vi "sub_InitDevices.vi"(8 "error in (no error)":errorcluster, 10 "Dynamic data":T1, 11 "Input parameters":T2={"Measurement type"=enum."Test", "Sensor type"=enum."One channel", "Input file"="", "Output file"="test.txt", "Open after execution?"=FALSE, "Display channel"=0, "Voltage Delay (s)"=0.5, "Switch Delay (s)"=0.01, "VISA resource name source"="", "VISA resource name LCR"="", "Voltage Limit (V)"=1000.0, "Enable Voltage Auto Range (T:Enable)"=TRUE, "Voltage Manual Range (1.0)"=1.0, "Compliance  Level (uA)"=10.0} {"Voltage Limit (V)" format="%#_13g"; "Voltage Delay (s)" format="%#_13g"; "Switch Delay (s)" format="%#_13g"}) -> (0 "error out":errorcluster, 2 "Dynamic data":T1, 3 "Input parameters":T2={"Measurement type"=enum."Test", "Sensor type"=enum."One channel", "Input file"="", "Output file"="test.txt", "Open after execution?"=FALSE, "Display channel"=0, "Voltage Delay (s)"=0.5, "Switch Delay (s)"=0.01, "VISA resource name source"="", "VISA resource name LCR"="", "Voltage Limit (V)"=1000.0, "Enable Voltage Auto Range (T:Enable)"=TRUE, "Voltage Manual Range (1.0)"=1.0, "Compliance  Level (uA)"=10.0} {"Voltage Limit (V)" format="%#_13g"; "Voltage Delay (s)" format="%#_13g"; "Switch Delay (s)" format="%#_13g"})   [LabVIEW 2015]
uses:
  Program Files (x86)/National Instruments/LabVIEW 2016/instr.lib/Keithley 24XX/Keithley 24XX.lvlib
  Input_parameters.ctl
  Dynamic_data.ctl
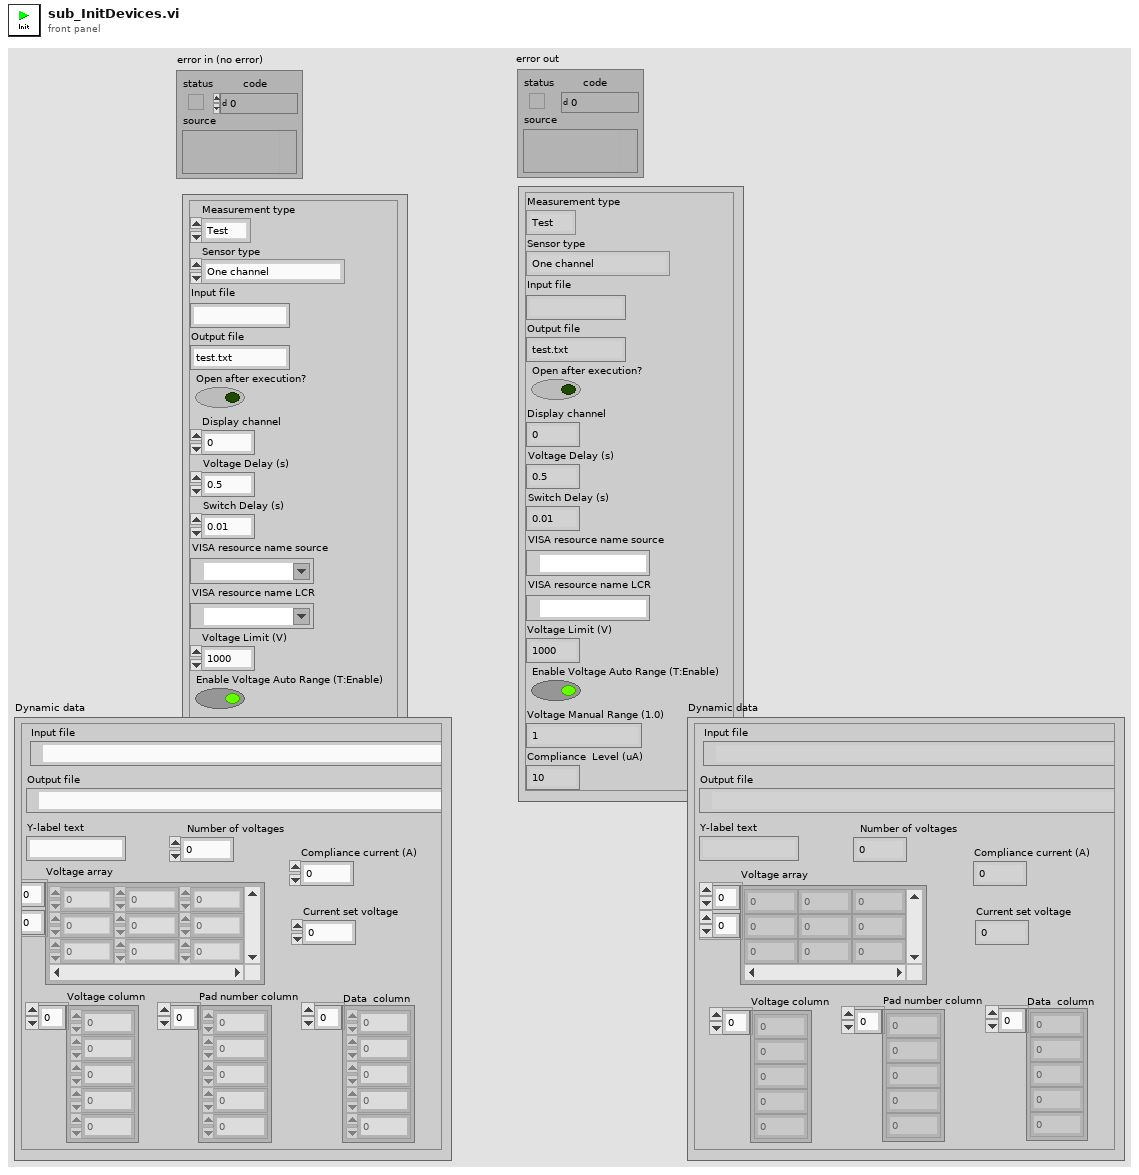
[diagram p1: front panel]
types:
  T1 = typedef "Dynamic_data.ctl" = cluster{"Input file":path, "Output file":path, "Y-label text":string, "Voltage array":dbl[][], "Current set voltage":dbl, "Voltage column":dbl[], "Pad number column":dbl[], "Data  column":dbl[], "Number of voltages":i32, "Compliance current (A)":dbl}
  T2 = typedef "Input_parameters.ctl" = cluster{"Measurement type":enum16{"IV", "CV", "Test"}, "Sensor type":enum16{"6''", "8''", "One channel"}, "Input file":string, "Output file":string, "Open after execution?":bool, "Display channel":i32, "Voltage Delay (s)":dbl, "Switch Delay (s)":dbl, "VISA resource name source":refnum<visa-resource-name>, "VISA resource name LCR":refnum<visa-resource-name>, "Voltage Limit (V)":dbl, "Enable Voltage Auto Range (T:Enable)":bool, "Voltage Manual Range (1.0)":dbl, "Compliance  Level (uA)":dbl}
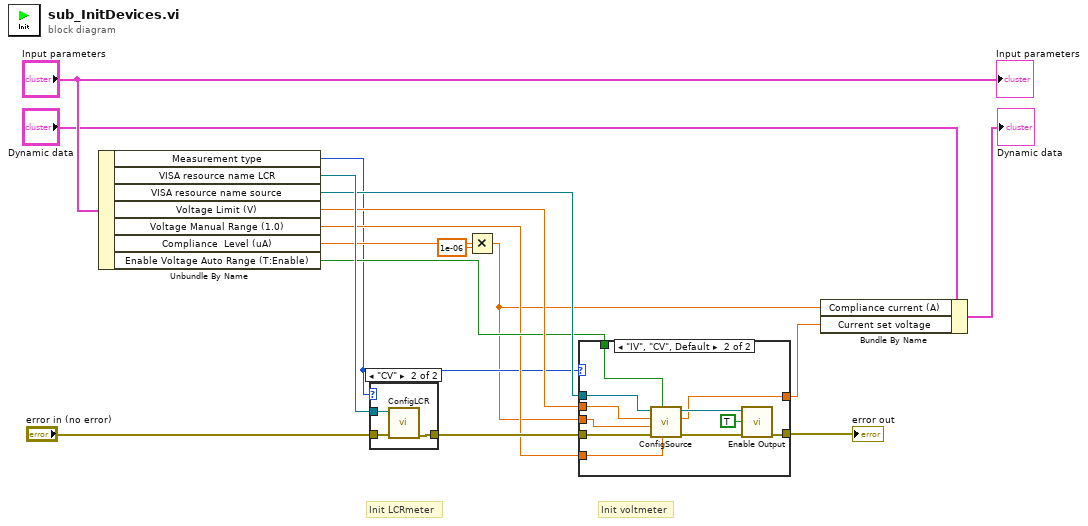
[diagram p0: block diagram]
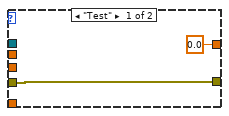
[diagram p2: hidden frame]
diagram:
  # "Init LCRmeter"
  # "Init voltmeter"
  n1 = Unbundle By Name("Input parameters") -> ("Measurement type"=w5:enum16{"IV", "CV", "Test"}, "VISA resource name LCR"=w12:refnum<visa-resource-name>, "VISA resource name source"=w11:refnum<visa-resource-name>, "Voltage Limit (V)"=w10:dbl, "Voltage Manual Range (1.0)"=w6:dbl, "Compliance  Level (uA)"=w8:dbl, "Enable Voltage Auto Range (T:Enable)"=w7:bool)
  n2 = case shown="\"CV\"" w5 {
    tunnel: "error in (no error)" -> [w17 w20]
    tunnel: [w17 w19] -> w14
    tunnel: w12 -> [_ w18]
    frame "IV", "Test", Default {
    }
    frame "CV" {
      n3 = call "ConfigLCR.vi"("VISA resource name LCR"=w18, "error in (no error)"=w20) -> ("error out"=w19:errorcluster)  [unwired: 12 in, 1 out]
    }
  }
  n4 = Multiply(x=w8, y=1e-06) -> (x*y=w1:dbl)
  n5 = case shown="\"IV\", \"CV\", Default" w5 {
    tunnel: [w22 w32] -> w13
    tunnel: w14 -> [w22 w29]
    tunnel: [0.0 ("Output Level (0)") w28] -> w2
    tunnel: w11 -> [_ w27]
    tunnel: w10 -> [_ w26]
    tunnel: w1 -> [_ w25]
    tunnel: w7 -> [_ w24]
    tunnel: w6 -> [_ w23]
    frame "Test" {
    }
    frame "IV", "CV", Default {
      n6 = call "ConfigSource.vi"("Voltage Manual Range (1.0)"=w23, "Single measurement? 2"=w24, "error in (no error)"=w29, "Compliance  Level (0.1)"=w25, "Voltage Limit (0.0 V)"=w26, "VISA resource name"=w27) -> ("error out"=w30:errorcluster, "Output Level (0)"=w28:dbl, "VISA resource name out"=w31:refnum<visa-resource-name>)  [unwired: 3 in]
      n7 = call "Enable Output.vi"("error in (no error)"=w30, "Enable Output (T: Enable)"=TRUE ("Enable Output"), "VISA resource name"=w31) -> ("error out"=w32:errorcluster)  [unwired: 7 in, 1 out]
    }
  }
  "error out" <- w13
  n8 = Bundle By Name(cluster="Dynamic data", "Compliance current (A)"=w1, "Current set voltage"=w2) -> (→"Dynamic data":T1)
  "Input parameters" <- "Input parameters"
